vi "16_Helper_Init.vi"(8 "Error In":errorcluster, 11 "reference in":refnum<class "16_Helper.lvclass"> caption="This control should only be used when\na sub class is inheriting this class") -> (0 "Error Out":errorcluster, 3 "reference out":refnum<class "16_Helper.lvclass"> caption="This indicator should only be used when\na sub class is inheriting this class")   [LabVIEW 2020, in "16_Helper.lvclass"]
uses:
  16_Helper.lvclass
  16_Helper.lvclass/16_Helper.ctl
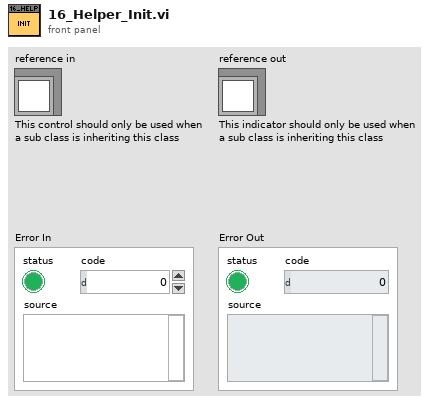
[diagram p1: front panel]
types:
  T1 = typedef "16_Helper.lvclass/ObjectAttributes.ctl" = cluster{"VersionNumberSum":u64}
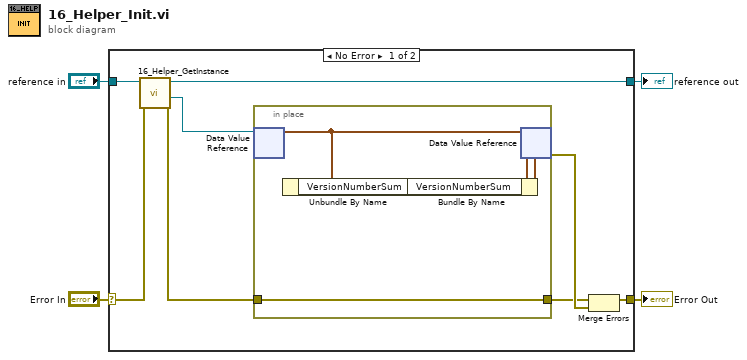
[diagram p0: block diagram]
diagram:
  n1 = case shown="No Error" "Error In" {
    selector: "Error In" -> [w10 w18]
    tunnel: [w11 w18] -> w3
    tunnel: "reference in" -> [w9 w17]
    tunnel: [w7 w17] -> w1
    frame No Error {
      n2 = call "16_Helper_GetInstance.vi"("error in"=w10, "reference in"=w9) -> ("error out"=w6:errorcluster, "DVRRefOut"=w8:refnum<data-value>, "reference out"=w7:refnum<class "16_Helper.lvclass">)  [unwired: 5 in, 2 out]
      n3 = in-place {
        in-place-border: w6 -> [w13]
        in-place-border: [w13] -> w5
        n4 = in-place-dvr #1(w8) -> (w15:T1)  [unwired: 1 out]
        n5 = Unbundle By Name(w15) -> ("VersionNumberSum"=w14:u64)
        n6 = Bundle By Name(cluster=w15, "VersionNumberSum"=w14) -> (w16:T1)
        n7 = in-place-dvr #1(w16) -> (w12:errorcluster)  [unwired: 1 out]
      }
      n8 = Merge Errors(w5, w12) -> (w11:errorcluster)
    }
    frame Error {
    }
  }
  "Error Out" <- w3
  "reference out" <- w1
